vi "mclamp_zero_VC_offset.vi"(8 "error in (no error)":errorcluster, 9 "set holding (mV)":dbl, 10 "Error in":i32, 11 "Multiclamp Handle Out":u32) -> (0 "error out":errorcluster, 2 "error out":i32)   [LabVIEW 2019]
uses:
  patcherBot_software_all/patcherBot_Software/patcherBot/AxMultiClampMsg.dll
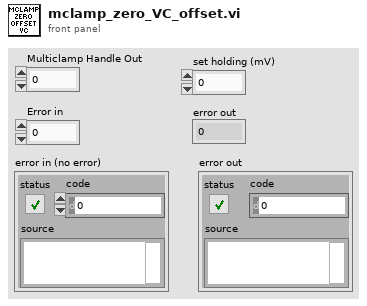
[diagram p1: front panel]
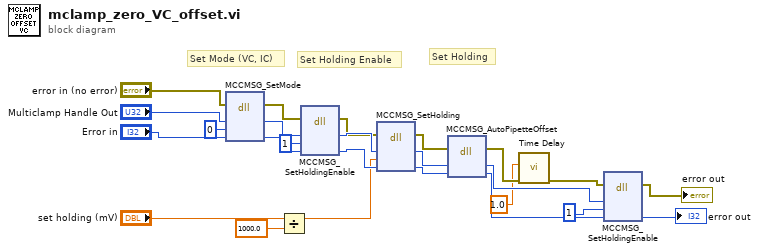
[diagram p0: block diagram]
diagram:
  # "Set Holding Enable"
  # "Set Holding"
  # "Set Mode (VC, IC)"
  n1 = dll-call lib="C:/Users/might/Dropbox (GaTech)/patcherBot_software_all/patcherBot_Software/patcherBot/AxMultiClampMsg.dll" fn="MCCMSG_SetMode"(error in="error in (no error)", "handle"="Multiclamp Handle Out", "ModeConstant"=u32 0, "error"="Error in") -> (error out=w14:errorcluster, "handle"=w12:u32, "error"=w13:i32)  [unwired: 4 in, 1 out]
  n2 = Divide(x="set holding (mV)", y=1000.0) -> (x/y=w2:dbl)
  n3 = dll-call lib="C:/Users/might/Dropbox (GaTech)/patcherBot_software_all/patcherBot_Software/patcherBot/AxMultiClampMsg.dll" fn="MCCMSG_SetHoldingEnable"(error in=w14, "handle"=w12, "ModeConstant"=1, "error"=w13) -> (error out=w15:errorcluster, "handle"=w17:u32, "error"=w16:i32)  [unwired: 4 in, 1 out]
  n4 = dll-call lib="C:/Users/might/Dropbox (GaTech)/patcherBot_software_all/patcherBot_Software/patcherBot/AxMultiClampMsg.dll" fn="MCCMSG_SetHolding"(error in=w15, "handle"=w17, "ModeConstant"=w2, "error"=w16) -> (error out=w21:errorcluster, "handle"=w19:u32, "error"=w20:i32)  [unwired: 4 in, 1 out]
  n5 = dll-call lib="C:/Users/might/Dropbox (GaTech)/patcherBot_software_all/patcherBot_Software/patcherBot/AxMultiClampMsg.dll" fn="MCCMSG_AutoPipetteOffset"(error in=w21, "handle"=w19, "error"=w20) -> (error out=w6:errorcluster, "handle"=w22:u32, "error"=w23:i32)  [unwired: 3 in, 1 out]
  n6 = call "Time Delay"("error in (no error)"=w6, "Delay Time (s)"=1.0) -> ("error out"=w5:errorcluster)  [unwired: 9 in]
  n7 = dll-call lib="C:/Users/might/Dropbox (GaTech)/patcherBot_software_all/patcherBot_Software/patcherBot/AxMultiClampMsg.dll" fn="MCCMSG_SetHoldingEnable"(error in=w5, "handle"=w22, "ModeConstant"=1, "error"=w23) -> (error out=→"error out":errorcluster, "error"=→"error out":i32)  [unwired: 5 in, 1 out]
